vi "New.vi"(8 "error in (no error)":errorcluster, 11 "reference in":refnum<class "Frequency_Counter_BK.lvclass">) -> (0 "error out":errorcluster, 3 "reference out":refnum<class "Frequency_Counter_BK.lvclass">)   [LabVIEW 2022 SP3, in "Frequency_Counter_BK.lvlib" / "Frequency_Counter_BK.lvclass"]
uses:
  Frequency_Counter_BK.lvclass
  ObjectAttributes.ctl
  Config.ctl
  Frequency_Counter_BK.lvclass/Frequency_Counter_BK.ctl
  Components/Frequency_Counter_Base.lvlibp/Frequency_Counter_Base.lvclass
panel:
  in  "Data":T1 {"Config"."Gate_Time" items=["0.01", "0.1", "1", "10"]; "Config"."Function" items=["Frequency A", "Frequency B", "Frequency C", "Period", "Total", "Ratio", "T.I"]}
  # "seconds"
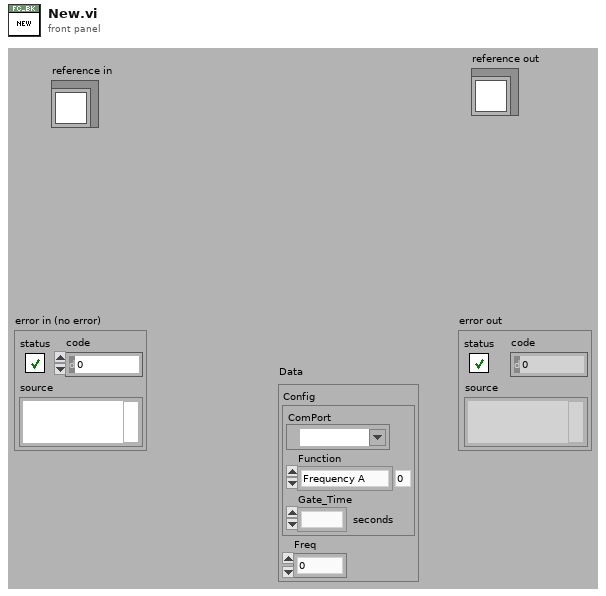
[diagram p1: front panel]
types:
  T1 = typedef "Frequency_Counter_BK.lvlib/Frequency_Counter_BK.lvclass/ObjectAttributes.ctl" = cluster{"Config":T2, "Freq":dbl}
  T2 = typedef "Frequency_Counter_BK.lvlib/Frequency_Counter_BK.lvclass/Config.ctl" = cluster{"ComPort":refnum<visa-resource-name>, "Function":i8, "Gate_Time":i8}
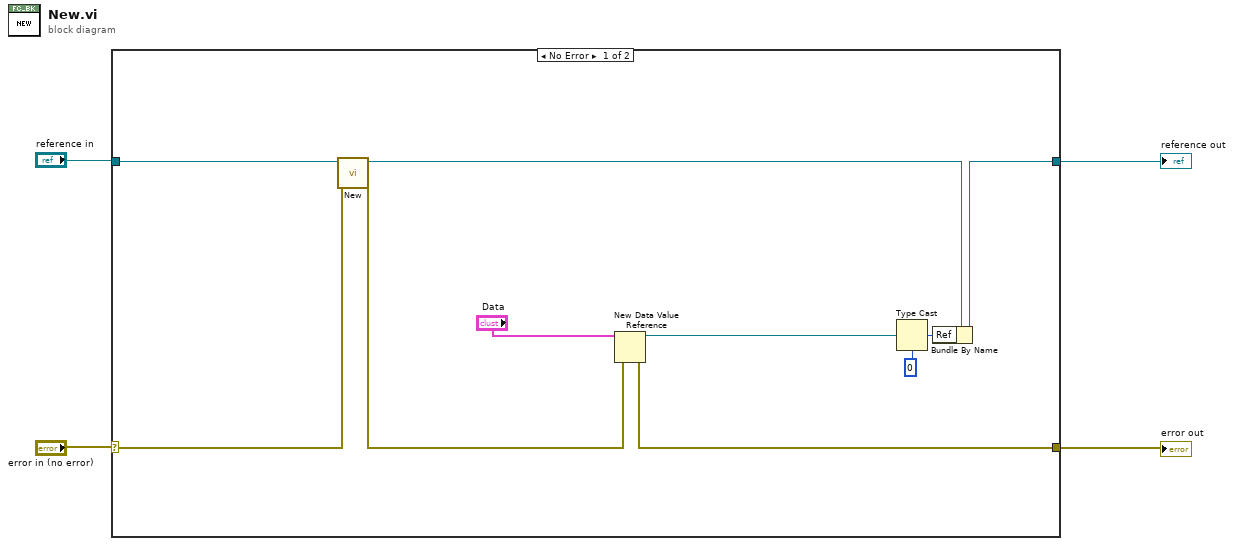
[diagram p0: block diagram]
diagram:
  n1 = case shown="No Error" "error in (no error)" {
    selector: "error in (no error)" -> [w6 w16]
    tunnel: [w7 w16] -> w2
    tunnel: "reference in" -> [w14 w15]
    tunnel: [w13 w15] -> w1
    frame No Error {
      n2 = call-parent "New.vi"("error in (no error)"=w6, "reference in"=w14) -> ("error out"=w5:errorcluster, "reference out"=w12:refnum<class "Frequency_Counter_BK.lvclass">)  [unwired: 8 in]
      n3 = New Data Value Reference(data value="Data", error in=w5) -> (data value reference=w10:refnum<data-value>, error out=w7:errorcluster)
      n4 = Type Cast(type=u32 0 ("DataRef"), x=w10) -> (*(type *) &x=w9:u32)
      n5 = Bundle By Name(cluster=w12, "Ref"=w9) -> (w13:refnum<class "Frequency_Counter_BK.lvclass">)
    }
    frame Error {
    }
  }
  "error out" <- w2
  "reference out" <- w1
